vi "LinearPlntInvFF_GetUff_Single.vi"(9 "Row":i32, 11 "Linear Plnt Inversion FF":T1) -> (3 "Uff":dbl)   [LabVIEW 2019, in "Trajectory_Library.lvlib"]
doc: "Returns an element of the previously calculated feedforward.\n \nInputs:\n - LinearPlntInversionFF -- system data cluster\n - row -- Row of uff.\n\nOutputs:\n - Uff -- The row of the calculated feedforward."
uses:
  Trajectory_Library.lvlib
  <vilib>/Analysis/Matrix/Datatypes/RealMatrix.ctl
  <vilib>/Analysis/Matrix/NI_Matrix.lvlib
  TypeDef/LINEAR_PLANT_INV_FF.ctl
panel:
  # "<States,1>"
  # "<Inputs,1>"
  # "<States,Inputs>"
  # "<States,States>"
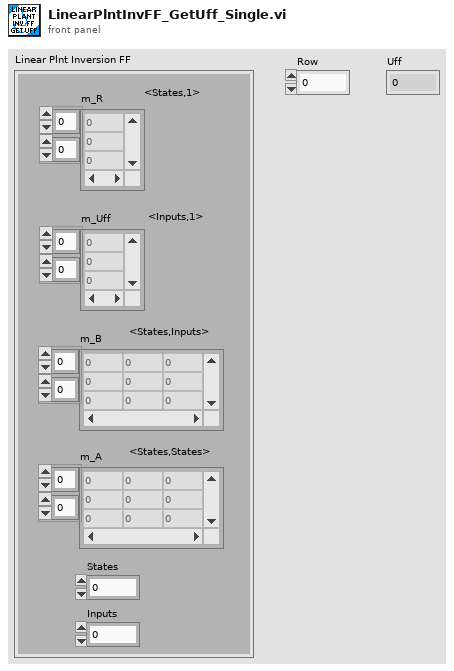
[diagram p1: front panel]
types:
  T1 = typedef "Trajectory_Library.lvlib/LINEAR_PLANT_INV_FF.ctl" = cluster{"m_R":T2, "m_Uff":T2, "m_B":T2, "m_A":T2, "States":i32, "Inputs":i32}
  T2 = typedef "NI_Matrix.lvlib/RealMatrix.ctl" = dbl[][]
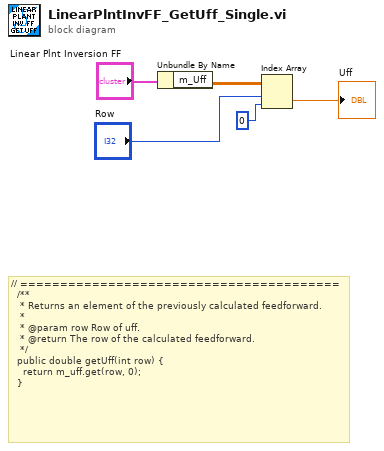
[diagram p0: block diagram]
diagram:
  # "// ========================================\n  /**\n   * Returns an element of the previously calculated feedforward.\n   *\n   * @param row Row of uff.\n   * @return The row of the calculated feedforward.\n   */\n  public double getUff(int row) {\n    return m_uff.get(row, 0);\n  }"
  n1 = Unbundle By Name("Linear Plnt Inversion FF") -> ("m_Uff"=w4:T2)
  n2 = Index Array(array=w4, index (row)="Row", index (col)=0) -> (element=→"Uff":dbl)
